vi "Set Marker.vi"(0 "GMaps API in":refnum<class "GMaps API.lvclass">, 1 "Marker":T1={"Marker Color"="", "Marker Size "="", "Marker Label"="", "Marker State"="", "Marker City"=" ", "Marker Street"=""}, 5 "error in (no error)":errorcluster) -> (14 "GMaps API out":refnum<class "GMaps API.lvclass">, 19 "error out":errorcluster)   [LabVIEW 2016, in "GMaps API.lvclass"]
doc: "Sets a set of one marker (map pins) at a set of location."
uses:
  GMaps API.lvclass
  Controls/Marker.ctl
  GMaps API.lvclass/GMaps API.ctl
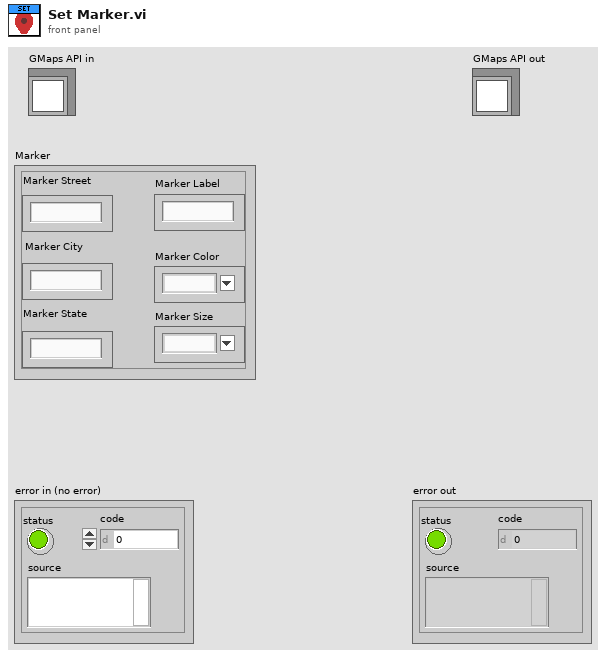
[diagram p1: front panel]
types:
  T1 = typedef "GMaps API.lvclass/Marker.ctl" = cluster{"Marker Color":string, "Marker Size ":string, "Marker Label":string, "Marker State":string, "Marker City":string, "Marker Street":string}
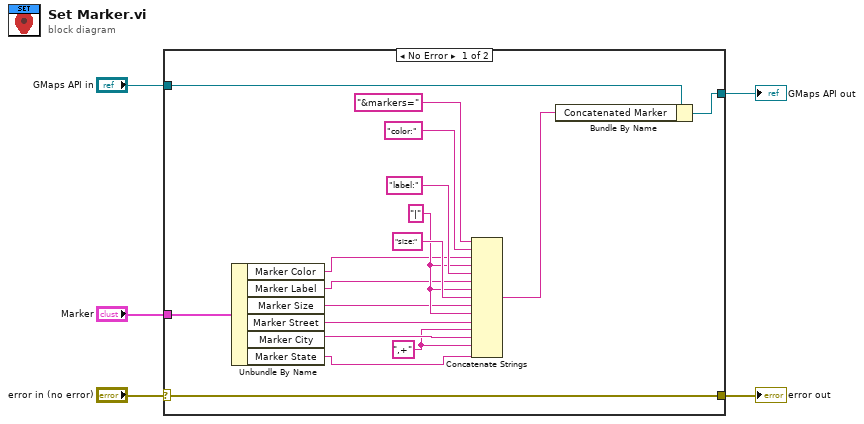
[diagram p0: block diagram]
diagram:
  n1 = case shown="No Error" "error in (no error)" {
    selector: "error in (no error)" -> [w22 w24]
    tunnel: [w22 w24] -> w4
    tunnel: [w21 w23] -> w2
    tunnel: "GMaps API in" -> [w6 w23]
    tunnel: "Marker" -> [w15 _]
    frame No Error {
      w8 = ",+" ("string")
      w16 = "|"
      n2 = Unbundle By Name(w15) -> ("Marker Color"=w9:string, "Marker Label"=w10:string, "Marker Size"=w11:string, "Marker Street"=w12:string, "Marker City"=w13:string, "Marker State"=w14:string)
      n3 = Concatenate Strings("&markers=", "color:", w9, w16, "label:", w10, w16, "size:", w11, w16, w12, w8, w13, w8, w14) -> (w7:string)
      n4 = Bundle By Name(cluster=w6, "Concatenated Marker"=w7) -> (w21:refnum<class "GMaps API.lvclass">)
    }
    frame Error {
    }
  }
  "error out" <- w4
  "GMaps API out" <- w2
